vi "Enqueue Single State.vi"(6 "Priority":T1, 8 "error in (no error)":errorcluster, 10 "String":string, 11 "QDMH in":refnum<class "QDMH.lvclass">) -> (0 "error out":errorcluster, 3 "QDMH out":refnum<class "QDMH.lvclass">)   [LabVIEW 2023, in "QDMH.lvlib" / "QDMH.lvclass"]
doc: "Enqueue Fully Formed message with data\nPriority determines if the item is enqueued at the end of the stack or the front:\n\nLow: Add to End\nHigh: Add to front"
uses:
  Library/QDMH.lvclass
  Custom Controls/Enqueue Priority.ctl
  Custom Controls/Message.ctl
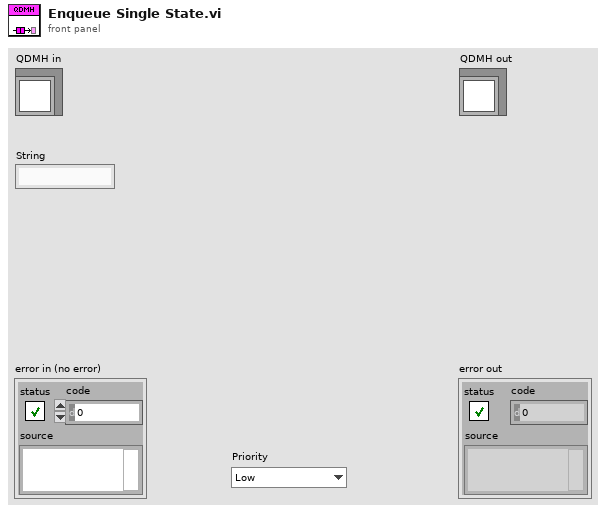
[diagram p1: front panel]
types:
  T1 = typedef "QDMH.lvlib/QDMH.lvclass/Enqueue Priority.ctl" = enum16{"Low", "High"}
  T2 = typedef "QDMH.lvlib/QDMH.lvclass/Message.ctl" = cluster{"State":string, "Data":variant}
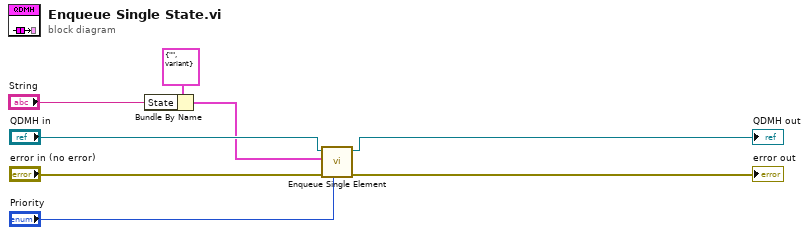
[diagram p0: block diagram]
diagram:
  n1 = Bundle By Name(cluster=T2 {"State"="", "Data"=variant} ("Message"), "State"="String") -> (w1:T2)
  n2 = call "Enqueue Single Element.vi"("Priority"="Priority", "error in (no error)"="error in (no error)", "Message"=w1, "QDMH in"="QDMH in") -> ("error out"=→"error out":errorcluster, "QDMH out"=→"QDMH out":refnum<class "QDMH.lvclass">)  [unwired: 6 in]
